vi "Parse SSH_FXP_VERSION.vi"(8 "error in":errorcluster, 11 "payload":u8[](array[numeric])) -> (0 "error out":errorcluster, 3 "extensions":set{T1}(c389))   [LabVIEW 2020, in "NI_SFTP.lvlib" / "Low Level Connection.lvclass"]
uses:
  <vilib>/net/SFTP/Low Level Connection/Low Level Connection.lvclass
  <vilib>/net/SFTP/Low Level Connection/Extension Pair.ctl
  f023bfa8-f8fb-3feb-c0fc-b0554016e43f.vi
  248d59e0-ee9f-3fd5-30f8-f80d1baee43f.vi
  <vilib>/net/SFTP/Low Level Connection/Assert Length.vi
  <vilib>/Bit Manipulation/Network-Order Bytes To Words Poly.vi
  <vilib>/Bit Manipulation/wrappers/Network-Order Bytes To Words/Network-Order Bytes To Words U32.vi
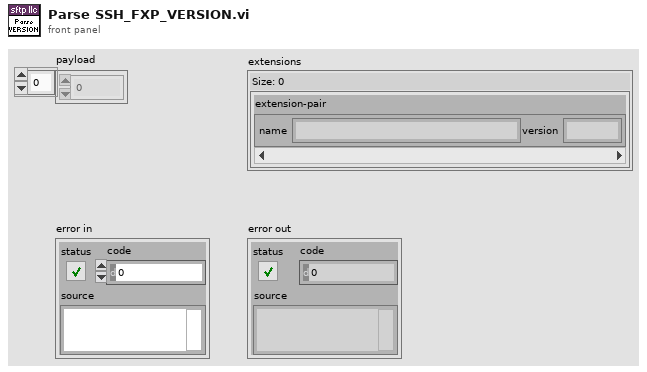
[diagram p1: front panel]
types:
  T1 = typedef "NI_SFTP.lvlib/Low Level Connection.lvclass/Extension Pair.ctl" = cluster{"name":string, "version":string}
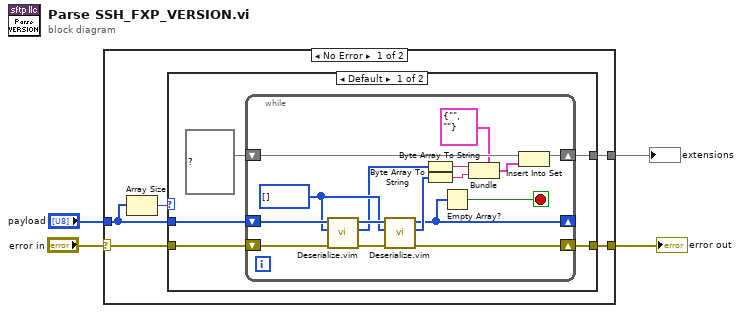
[diagram p0: block diagram]
diagram:
  n1 = case shown="No Error" "error in" {
    selector: "error in" -> [w6 w32]
    tunnel: [w7 w32] -> w3
    tunnel: "payload" -> [w9 _]
    tunnel: [w5 _] -> w1
    frame No Error {
      n2 = Array Size(array=w9) -> (size(s)=w8:i32)
      n3 = case shown="Default" w8 {
        tunnel: w9 -> [w14 _]
        tunnel: w6 -> [w13 w31]
        tunnel: [w12 w31] -> w7
        tunnel: [w11 _] -> w5
        frame Default {
          n4 = while {
            shift-right: [w20] -> _
            shift-left: w14 -> [w30]
            shift-right: [w26] -> w12
            shift-left: w13 -> [w28]
            shift-right: [w25] -> w11
            shift-left: set{T1} {} ("extensions") -> [w17]
            stop <- w21 stop-if-true
            w24 = u8[] [] ("payload")
            n5 = call "Deserialize.vim"("error in"=w28, "type"=w24, "bytes"=w30) -> ("error out"=w27:errorcluster, "value"=w23:u8[], "remaining bytes"=w29:u8[])  [unwired: 6 in]
            n6 = call "Deserialize.vim"("error in"=w27, "type"=w24, "bytes"=w29) -> ("error out"=w26:errorcluster, "value"=w22:u8[], "remaining bytes"=w20:u8[])  [unwired: 6 in]
            n7 = Byte Array To String(unsigned byte array=w23) -> (string=w19:string)
            n8 = Byte Array To String(unsigned byte array=w22) -> (string=w18:string)
            n9 = Empty Array?(array=w20) -> (empty?=w21:bool)
            n10 = Bundle(cluster=T1 {"name"="", "version"=""} ("extension-pair"), "name"=w19, "version"=w18) -> (w16:T1)
            n11 = Insert Into Set(10:w16, 11:w17) -> (3:w25:set{T1})  [unwired: 1 out]
          }
        }
        frame 0 {
        }
      }
    }
    frame Error {
    }
  }
  "error out" <- w3
  "extensions" <- w1
